vi "Wait for Operation Complete.vi"(8 "error in (no error)":errorcluster, 9 "Maximum Time (2000ms)":u32=2000, 11 "VISA resource name":refnum<visa-resource-name>) -> (0 "error out":errorcluster, 3 "VISA resource name out":refnum<visa-resource-name>)   [LabVIEW 2015, in "Tektronix 7000 Series.lvlib"]
doc: "Waits for the instrument to complete the execution of all pending operations.\n\n<B>Note:</B> \nThis VI does not check the status of an instrument."
uses:
  Tektronix 7000 Series.lvlib
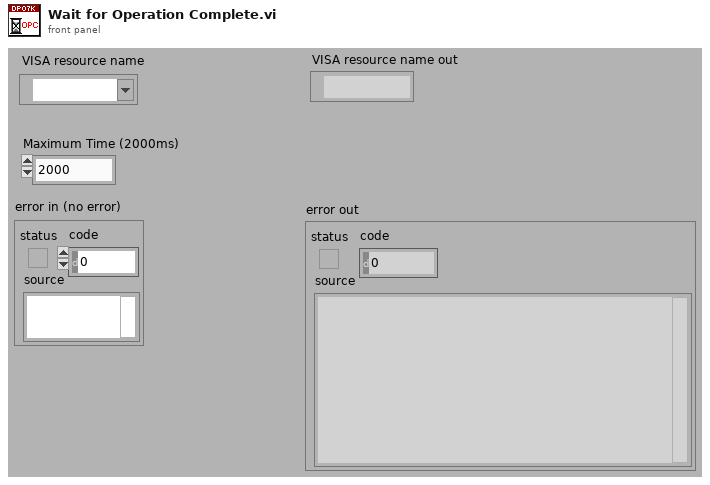
[diagram p1: front panel]
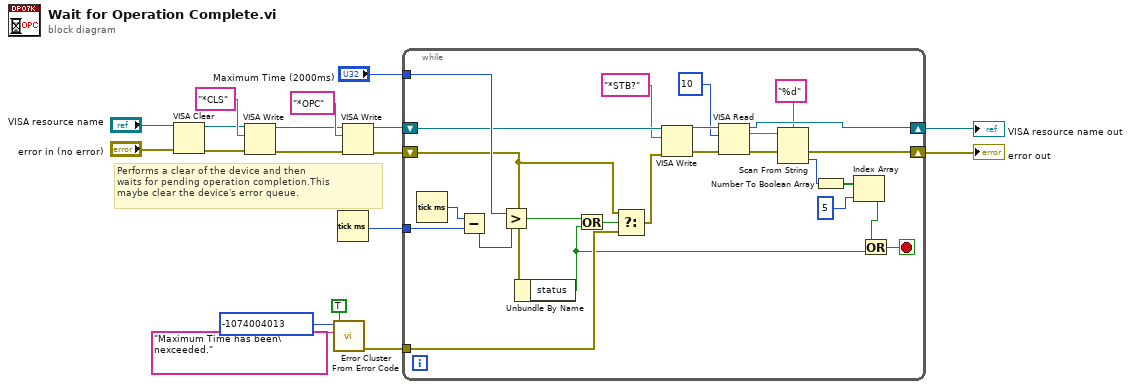
[diagram p0: block diagram]
diagram:
  # "Performs a clear of the device and then \nwaits for pending operation completion.This \nmaybe clear the device's error queue."
  n1 = VISA Clear(VISA resource name="VISA resource name", error in (no error)="error in (no error)") -> (VISA resource name out=w4:refnum<visa-resource-name>, error out=w3:errorcluster)
  n2 = VISA Write(VISA resource name=w4, write buffer="*CLS", error in (no error)=w3) -> (VISA resource name out=w2:refnum<visa-resource-name>, error out=w1:errorcluster)  [unwired: 1 out]
  n3 = call <vilib>:"Error Cluster From Error Code.vi"("show call chain? (False)"=TRUE, "error message (\"\")"="Maximum Time has been\nexceeded." ("error message (\"\")"), "error code (0)"=-1074004013) -> ("error out"=w8:errorcluster)  [unwired: 6 in]
  n4 = Tick Count (ms)() -> (millisecond timer value=w13:u32)
  n5 = VISA Write(VISA resource name=w2, write buffer="*OPC", error in (no error)=w1) -> (VISA resource name out=w15:refnum<visa-resource-name>, error out=w14:errorcluster)  [unwired: 1 out]
  n6 = while {
    tunnel: w13 -> [w40]
    tunnel: "Maximum Time (2000ms)" -> [w36]
    tunnel: w8 -> [w33]
    shift-right: [w23] -> w7
    shift-left: w15 -> [w30]
    shift-right: [w19] -> w6
    shift-left: w14 -> [w32]
    stop <- w38 stop-if-true
    n7 = Tick Count (ms)() -> (millisecond timer value=w41:u32)
    n8 = Subtract(x=w41, y=w40) -> (x-y=w37:u32)
    n9 = Greater?(x=w36, y=w37) -> (0:w35:bool)
    n10 = Unbundle By Name(w32) -> ("status"=w31:bool)
    n11 = Or(x=w35, y=w31) -> (x .or. y?=w34:bool)
    n12 = Select(t=w32, s=w34, f=w33) -> (s? t:f=w29:errorcluster)
    n13 = VISA Write(VISA resource name=w30, write buffer="*STB?", error in (no error)=w29) -> (VISA resource name out=w27:refnum<visa-resource-name>, error out=w26:errorcluster)  [unwired: 1 out]
    n14 = VISA Read(VISA resource name=w27, byte count=u32 10, error in (no error)=w26) -> (VISA resource name out=w23:refnum<visa-resource-name>, read buffer=w22:string, error out=w24:errorcluster)  [unwired: 1 out]
    n15 = Scan From String(format string="%d", input string=w22, error in=w24) -> (error out=w19:errorcluster, output 1=w20:i32)  [unwired: 2 in, 2 out]
    n16 = Number To Boolean Array(number=w20) -> (Boolean array=w43:bool[])
    n17 = Index Array(array=w43, index=5) -> (element=w39:bool)
    n18 = Or(x=w39, y=w31) -> (x .or. y?=w38:bool)
  }
  "VISA resource name out" <- w7
  "error out" <- w6
